vi "capCalc_volProtPara.vi"(11 "volProtTri":dbl[](array[numeric])) -> (1 "signStart":i32, 2 "signLength":dbl, 3 "sigReps":i32)   [LabVIEW 2021]
uses:
  <vilib>/Analysis/baseanly.llb/Mean (DBL).vi
  <vilib>/Analysis/NI_AALBase.lvlib
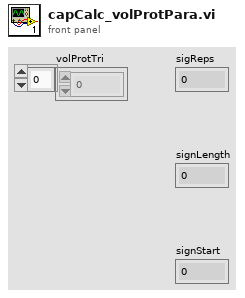
[diagram p1: front panel]
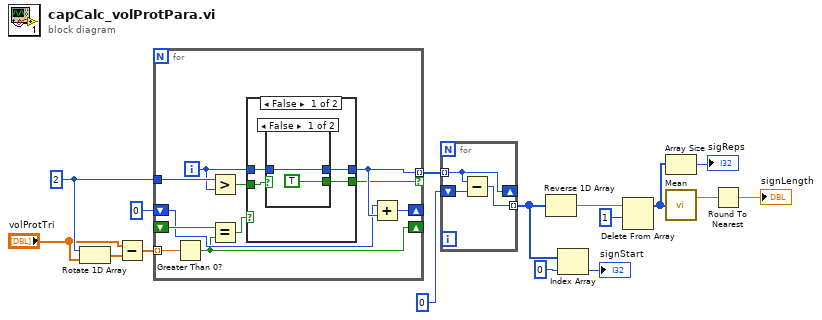
[diagram p0: block diagram]
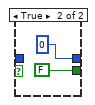
[diagram p2: hidden frame]
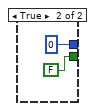
[diagram p3: hidden frame]
diagram:
  w3 = 2 ("n")
  n1 = Rotate 1D Array(1:"volProtTri", 2:w3) -> (0:w1:dbl[])
  n2 = Subtract(x="volProtTri", y=w1) -> (x-y=w16:dbl[])
  n3 = for {
    tunnel: w16 -> [w27] mode=indexing
    shift-right: [w18] -> _
    shift-left: _ -> [w26]
    tunnel: [w25] -> w5 mode=indexing if=w17
    shift-right: [w24] -> _
    shift-left: 0 -> [w20]
    tunnel: w3 -> [w23]
    i -> [w19]
    n4 = Greater Than 0?(x=w27) -> (x > 0?=w18:bool)
    n5 = Greater?(x=w23, y=w19) -> (0:w21:bool)
    n6 = Equal?(x=w26, y=w18) -> (x = y?=w22:bool)
    n7 = case shown="False" w22 {
      tunnel: [w31 0] -> w25
      tunnel: w21 -> [w30 _]
      tunnel: w19 -> [w29 _]
      tunnel: [w28 FALSE] -> w17
      frame False {
        n8 = case shown="False" w30 {
          tunnel: [w33 0] -> w31
          tunnel: w29 -> [w33 _]
          tunnel: [TRUE FALSE] -> w28
          frame False {
          }
          frame True {
          }
        }
      }
      frame True {
      }
    }
    n9 = Add(x=w20, y=w25) -> (x+y=w24:i32)
  }
  n10 = for {
    tunnel: w5 -> [w38] mode=indexing
    shift-right: [w38] -> _
    shift-left: 0 -> [w40]
    tunnel: [w39] -> w14 mode=indexing
    n11 = Subtract(x=w38, y=w40) -> (x-y=w39:i32)
  }
  n12 = Reverse 1D Array(array=w14) -> (reversed array=w13:i32[])
  n13 = Index Array(array=w14, index=0) -> (element=→"signStart":i32)
  n14 = Delete From Array(array=w13, length=1) -> (array with subset deleted=w9:i32[])  [unwired: 1 in, 1 out]
  n15 = Array Size(array=w9) -> (size(s)=→"sigReps":i32)
  n16 = call-poly <vilib>:"Mean.vi"("X"=w9) -> ("mean"=w7:dbl)  [unwired: 1 out]
  n17 = Round To Nearest(number=w7) -> (nearest integer value=→"signLength":dbl)
